vi "HEAD.vi"(6 "timeout (10000)":i32=10000, 8 "error in (no error)":errorcluster, 10 "url":string, 11 "HTTP Client Base in":refnum<class "HTTP Client Base.lvclass">) -> (0 "error out":errorcluster, 2 "headers":string, 3 "HTTP Client Base out":refnum<class "HTTP Client Base.lvclass">)   [LabVIEW 2021, in "HTTP Client Base.lvclass"]
uses:
  HTTP Client Base.lvclass
  HTTP Client Base.lvclass/HTTP Client Base.ctl
  <vilib>/httpClient/LabVIEWHTTPClient.lvlib
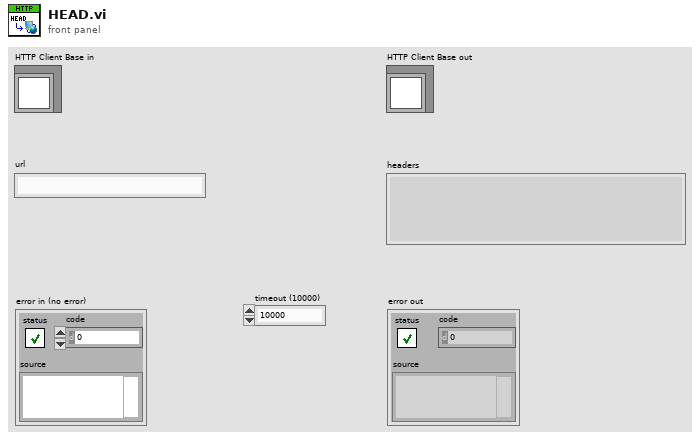
[diagram p1: front panel]
types:
  T1 = typedef "LabVIEWHTTPClient.lvlib/ClientHandle.ctl" = refnum<k1>
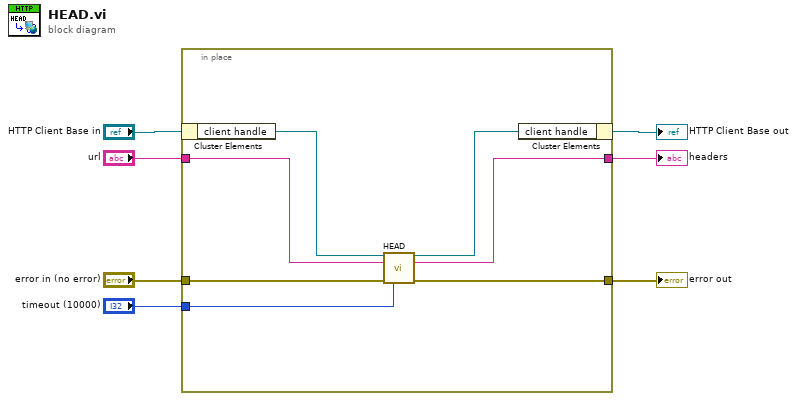
[diagram p0: block diagram]
diagram:
  n1 = in-place {
    in-place-border: "error in (no error)" -> [w14]
    in-place-border: [w13] -> w5
    in-place-border: "url" -> [w10]
    in-place-border: [w9] -> w2
    in-place-border: "timeout (10000)" -> [w8]
    n2 = in-place-cluster #1("HTTP Client Base in") -> ("client handle"=w12:T1)
    n3 = call <vilib>:"HEAD.vi"("client handle"=w12, "url"=w10, "error in (no error)"=w14, "timeout (10000)"=w8) -> ("client handle out"=w11:T1, "headers"=w9:string, "error out"=w13:errorcluster)  [unwired: 9 in]
    n4 = in-place-cluster #1("client handle"=w11) -> (→"HTTP Client Base out":refnum<class "HTTP Client Base.lvclass">)
  }
  "error out" <- w5
  "headers" <- w2
